vi "Unregister Sessions Impl.vi"(8 "error in":errorcluster, 11 "data in":T1) -> (0 "error out":errorcluster, 3 "data out":T1)   [LabVIEW 2020, in "MeasurementLink Session Management.lvlib" / "Session Reservation.lvclass"]
uses:
  Session Reservation.lvclass
  MeasurementLink gRPC Utilities/gRPC Client Pool/FGV Action.ctl
  MeasurementLink gRPC Utilities/gRPC Client Pool/gRPC Client Pool.lvclass
  MeasurementLink Session Management Client/RPC Messages/ni_measurementlink_sessionmanagement_v1_ChannelMapping.ctl
  MeasurementLink Session Management Client/MeasurementLink Session Management Client.lvlib
  MeasurementLink Session Management Client/RPC Messages/nidevice_grpc_Session.ctl
  MeasurementLink Session Management Client/RPC Messages/ni_measurementlink_sessionmanagement_v1_SessionInformation.ctl
  MeasurementLink Session Management Client/RPC Messages/ni_measurementlink_sessionmanagement_v1_UnregisterSessionsRequest.ctl
  MeasurementLink Instrument/IInstrument/IInstrument.lvclass
  Session and Driver Info.ctl
  MeasurementLink Session Management Client/RPC Messages/ni_measurementlink_PinMapContext.ctl
  Connection Map/Connection Map.lvclass
  IState/IState.lvclass
  Data.ctl
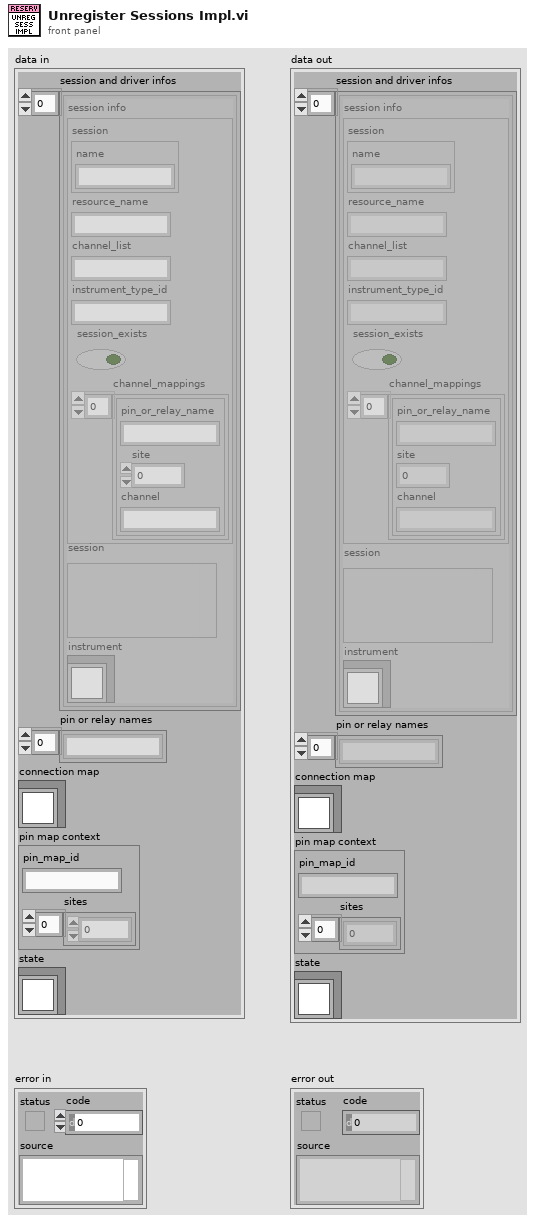
[diagram p1: front panel]
types:
  T1 = typedef "MeasurementLink Session Management.lvlib/Session Reservation.lvclass/Data.ctl" = cluster{"session and driver infos":T2[], "pin or relay names":string[], "connection map":refnum<class "Connection Map.lvclass">, "pin map context":T6, "state":refnum<class "IState.lvclass">}
  T2 = typedef "MeasurementLink Session Management.lvlib/Session Reservation.lvclass/Session and Driver Info.ctl" = cluster{"session info":T3, "session":variant, "instrument":refnum<class "IInstrument.lvclass">}
  T3 = typedef "MeasurementLink Session Management Client.lvlib/ni_measurementlink_sessionmanagement_v1_SessionInformation.ctl" = cluster{"session":T4, "resource_name":string, "channel_list":string, "instrument_type_id":string, "session_exists":bool, "channel_mappings":T5[]}
  T4 = typedef "MeasurementLink Session Management Client.lvlib/nidevice_grpc_Session.ctl" = cluster{"name":string}
  T5 = typedef "MeasurementLink Session Management Client.lvlib/ni_measurementlink_sessionmanagement_v1_ChannelMapping.ctl" = cluster{"pin_or_relay_name":string, "site":i32, "channel":string}
  T6 = typedef "MeasurementLink Session Management Client.lvlib/ni_measurementlink_PinMapContext.ctl" = cluster{"pin_map_id":string, "sites":i32[]}
  T7 = typedef "MeasurementLink Session Management Client.lvlib/ni_measurementlink_sessionmanagement_v1_UnregisterSessionsRequest.ctl" = cluster{"sessions":T3[]}
  T8 = typedef "MeasurementLink gRPC Utilities.lvlib/gRPC Client Pool.lvclass/FGV Action.ctl" = enum16{"Get Discovery Client", "Get Session Client", "Get Pinmap Client", "Destroy Clients"}
  T9 = typedef "grpc-lvsupport-release.lvlib/grpcId.ctl" = u64
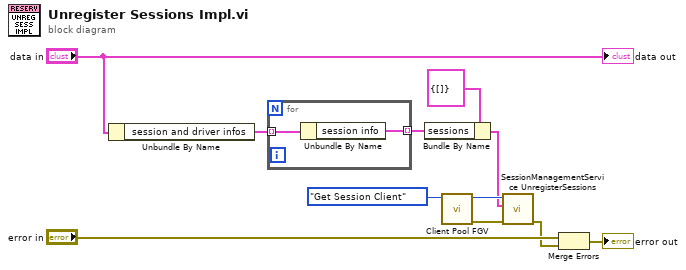
[diagram p0: block diagram]
diagram:
  n1 = Unbundle By Name("data in") -> ("session and driver infos"=w4:T2[])
  n2 = for {
    tunnel: w4 -> [w13] mode=indexing
    tunnel: [w12] -> w6 mode=indexing
    n3 = Unbundle By Name(w13) -> ("session info"=w12:T3)
  }
  n4 = Bundle By Name(cluster=T7 {"sessions"=[]} ("Request Data"), "sessions"=w6) -> (w5:T7)
  n5 = call "Client Pool FGV.vi"("Action"=FGV_Action."Get Session Client") -> ("error out"=w9:errorcluster, "grpc client id"=w8:T9)  [unwired: 9 in]
  n6 = call "SessionManagementService UnregisterSessions.vi"("error in"=w9, "Request Data"=w5, "gRPC ID"=w8) -> ("error out"=w2:errorcluster)  [unwired: 6 in, 2 out]
  n7 = Merge Errors("error in", w2) -> (→"error out":errorcluster)
  "data out" <- "data in"
